vi "GET Channels.vi"(7 "Channel Direction":string, 8 "error in (no error)":errorcluster, 11 "Item Ref in":T1 format="%.0x") -> (0 "error out":errorcluster, 3 "VS Channel Array":refnum<class "ChannelVS.lvclass">[](array[class]))   [LabVIEW 2021, in "Shared Variables CD 2.0 Configuration.lvlib" / "ChannelVS.lvclass"]
uses:
  ChannelVS.lvclass
  ChannelVS.lvclass/ChannelVS.ctl
  <vilib>/NI VeriStand/Custom Device API/Custom Device API.lvlib
  <vilib>/NI VeriStand/Custom Device API/Get Item Property (String).vi
  Shared/SV Global.vi
  <vilib>/NI VeriStand/Custom Device API/Get Item Property (Variant).vi
  OneDrive - NI/Documents/GitHub/Shared-Variable-Custom-Device-2.0/Modules/Channel.lvlibp/Channel.lvclass
  OneDrive - NI/Documents/GitHub/Shared-Variable-Custom-Device-2.0/Modules/Channel.lvlibp/1abvi3w/vi.lib/Utility/Data Type/Type Definitions/Data Type.ctl
  OneDrive - NI/Documents/GitHub/Shared-Variable-Custom-Device-2.0/Modules/Channel.lvlibp/1abvi3w/vi.lib/Utility/Data Type/NI_Data Type.lvlib
  <vilib>/NI VeriStand/Custom Device API/Custom Device Item Ref.ctl
  C:/Users/NPowley/OneDrive - NI/Documents/GitHub/Shared-Variable-Custom-Device-2.0/Modules/Channel.lvlibp/Channel.lvclass
  C:/Users/NPowley/Downloads/Shared-Variable-Custom-Device-2.0-master (8)/Shared-Variable-Custom-Device-2.0-master/Source_2017/Source/Shared Variables CD 2.0/Configuration/Support/ChannelVS/ChannelVS.lvclass
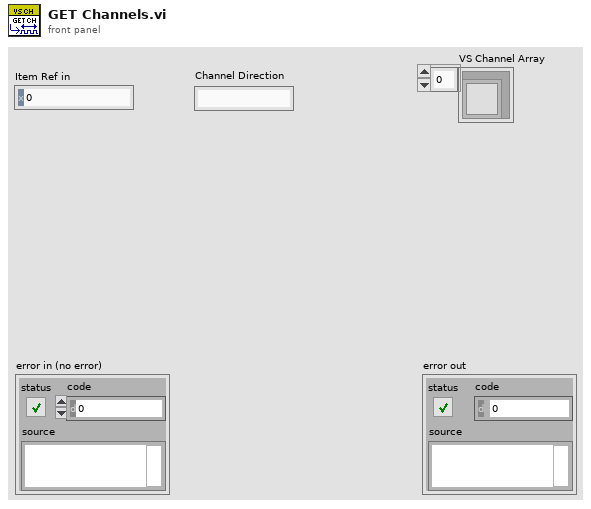
[diagram p1: front panel]
types:
  T1 = typedef "Custom Device API.lvlib/Custom Device Item Ref.ctl" = u64
  T2 = typedef "Channel.lvlibp/NI_Data Type.lvlib/Data Type.ctl" = enum8{"Invalid Type", "Void", "I8", "I16", "I32", "I64", "U8", "U16", "U32", "U64", "Single Float", "Double Float", "Extended Float", "Single Complex", "Double Complex", "Extended Complex", "Enum U8", "Enum U16", "Enum U32", "Enum U64", "Single Float With Unit", "Double Float With Unit", "Extended Float With Unit", "Single Complex with Unit", "Double Complex with Unit", "Extended Complex with Unit", "Boolean", "String", "Path", "Picture", "Tag", "Array", "Cluster", "Variant", "LV Variant", "Waveform", "Timestamp", "Digital Waveform", "Digital Data", "ExpressData", "Refnum", "External Data", "VI", "Poly VI", "LabVIEW Class Instance", "Fixed Point", "Set Collection", "Map Collection"}
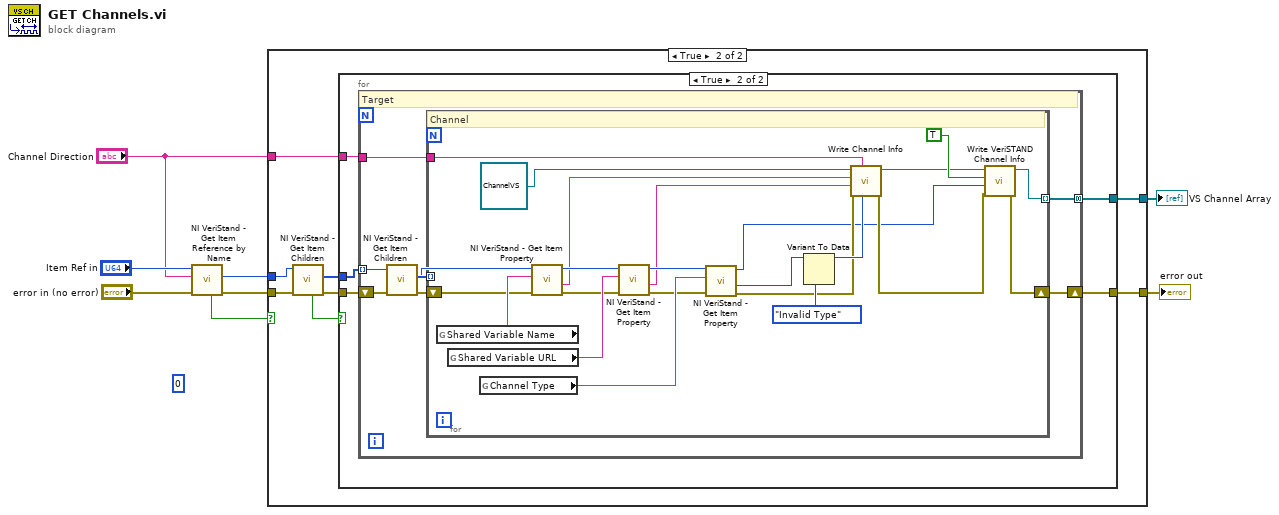
[diagram p0: block diagram]
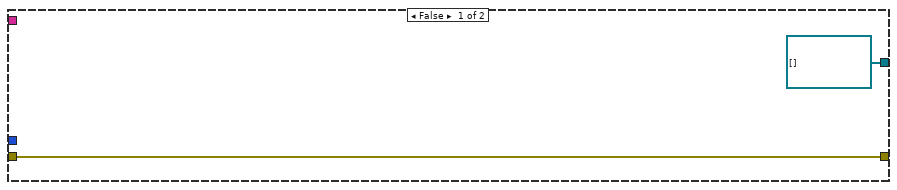
[diagram p2: hidden frame]
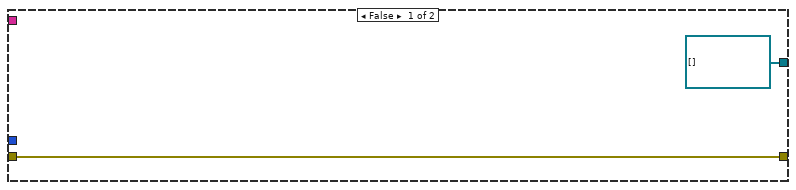
[diagram p3: hidden frame]
diagram:
  (unwired) T1 0 ("Item Ref in")
  n1 = call <vilib>:"NI VeriStand - Get Item Reference by Name.vi"("error in (no error)"="error in (no error)", "Item Name"="Channel Direction", "Parent Ref in"="Item Ref in") -> ("error out"=w5:errorcluster, "Item Ref"=w4:T1, "Found"=w2:bool)  [unwired: 5 in, 1 out]
  n2 = case shown="True" w2 {
    tunnel: [w10 w18] -> w8
    tunnel: [refnum<class "ChannelVS.lvclass">[] [] w15] -> w1
    tunnel: w5 -> [w10 w14]
    tunnel: w4 -> [_ w13]
    tunnel: "Channel Direction" -> [_ w12]
    frame False {
    }
    frame True {
      n3 = call <vilib>:"NI VeriStand - Get Item Children.vi"("error in (no error)"=w14, "Item Ref in"=w13) -> ("error out"=w17:errorcluster, "Child Refs"=w16:T1[], "Found"=w11:bool)  [unwired: 6 in, 1 out]
      n4 = case shown="True" w11 {
        tunnel: [w20 w25] -> w18
        tunnel: w17 -> [w20 w24]
        tunnel: w16 -> [_ w23]
        tunnel: [refnum<class "ChannelVS.lvclass">[] [] w22] -> w15
        tunnel: w12 -> [_ w21]
        frame False {
        }
        frame True {
          n5 = for {
            tunnel: w23 -> [w32] mode=indexing
            shift-right: [w28] -> w25
            shift-left: w24 -> [w30]
            tunnel: [w27] -> w22 mode=concatenating
            tunnel: w21 -> [w26]
            # "Target"
            n6 = call <vilib>:"NI VeriStand - Get Item Children.vi"("error in (no error)"=w30, "Item Ref in"=w32) -> ("error out"=w29:errorcluster, "Child Refs"=w31:T1[])  [unwired: 6 in, 2 out]
            n7 = for {
              tunnel: w31 -> [w36] mode=indexing
              shift-right: [w37] -> w28
              shift-left: w29 -> [w50]
              tunnel: [w39] -> w27 mode=indexing
              tunnel: w26 -> [w44]
              # "Channel"
              n8 = global read "SV Global.vi" "Shared Variable Name"() -> (w55:string)
              n9 = global read "SV Global.vi" "Shared Variable URL"() -> (w53:string)
              n10 = global read "SV Global.vi" "Channel Type"() -> (w52:string)
              n11 = call-poly <vilib>:"NI VeriStand - Get Item Property.vi"("error in (no error)"=w50, "Property Name"=w55, "Item Ref in"=w36) -> ("error out"=w49:errorcluster, "Value"=w46:string, "Item Ref out"=w54:T1)  [unwired: 5 in, 1 out]
              n12 = call-poly <vilib>:"NI VeriStand - Get Item Property.vi"("error in (no error)"=w49, "Property Name"=w53, "Item Ref in"=w54) -> ("error out"=w48:errorcluster, "Value"=w45:string, "Item Ref out"=w51:T1)  [unwired: 5 in, 1 out]
              n13 = call-poly <vilib>:"NI VeriStand - Get Item Property.vi"("error in (no error)"=w48, "Property Name"=w52, "Item Ref in"=w51) -> ("error out"=w40:errorcluster, "Value"=w47:variant, "Item Ref out"=w35:T1)  [unwired: 5 in, 1 out]
              n14 = Variant To Data(type=Data_Type."Invalid Type" ("DataType"), Variant=w47) -> (data=w42:T2)  [unwired: 1 in, 1 out]
              n15 = call "Write Channel Info.vi"("DataType"=w42, "Read or Write"=w44, "error in (no error)"=w40, "URL"=w45, "Name"=w46, "Channel in"=refnum<class "ChannelVS.lvclass"> refnum ("Shared Variables CD 2.0 Configuration.lvlib:ChannelVS.lvclass")) -> ("error out"=w38:errorcluster, "Channel out"=w33:refnum<class "ChannelVS.lvclass">)  [unwired: 4 in]
              n16 = call "Write VeriSTAND Channel Info.vi"("error in (no error)"=w38, "VeriSTAND Reference"=w35, "Exist in VeriSTAND"=TRUE, "ChannelVS in"=w33) -> ("error out"=w37:errorcluster, "ChannelVS out"=w39:refnum<class "ChannelVS.lvclass">)  [unwired: 6 in]
            }
          }
        }
      }
    }
  }
  "error out" <- w8
  "VS Channel Array" <- w1
